vi "Show Image Window.vi"   [LabVIEW 2020, in "g_ar_toolkit.image.lvlib"]
doc: "Show the Image in a named Image Window.\n\nNo user-interaction API is provided as these Windows are intended for debugging only."
uses:
  g_ar_toolkit.image.lvlib
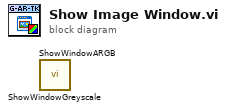
[diagram p0: block diagram]
diagram:
  n1 = call "ShowWindowGreyscale.vi"() -> ()  [unwired: 10 in, 2 out]
  n2 = call "ShowWindowARGB.vi"() -> ()  [unwired: 10 in, 2 out]
